vi "DN4_BufferedAO_SetData.vi"(7 "data in(DDT)":dynamicdata(waveform), 8 "error in (no error)":errorcluster, 9 "count":i32, 11 "Task ID":u32) -> (0 "error out":errorcluster, 2 "remaining count":i32, 3 "Task ID":u32)   [LabVIEW 2009]
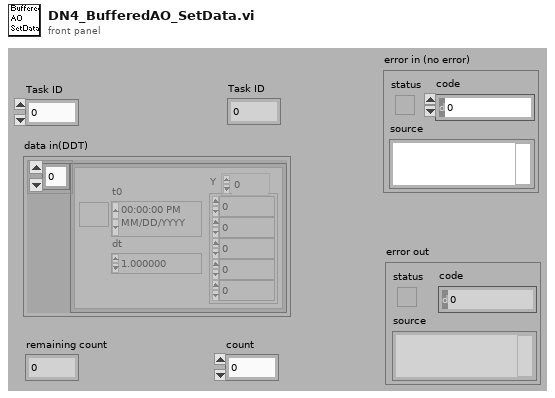
[diagram p1: front panel]
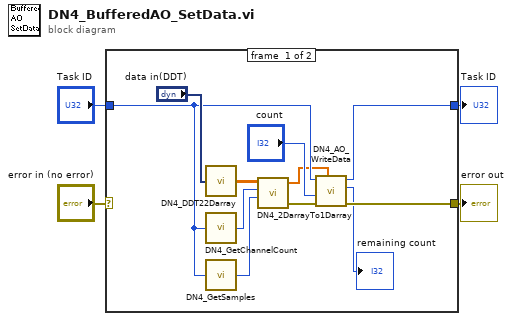
[diagram p0: block diagram]
diagram:
  n1 = case shown="No Error" "error in (no error)" {
    selector: "error in (no error)" -> [_ w17]
    tunnel: [w10 w16] -> w3
    tunnel: [w9 w17] -> w2
    tunnel: "Task ID" -> [w8 w16]
    frame #0 {
      n2 = call <userlib>:"DN4_DDT22Darray.vi"("data"="data in(DDT)") -> ("Array"=w14:dbl[][])
      n3 = call <userlib>:"DN4_GetChannelCount.vi"("Task ID"=w8) -> ("return type"=w13:i32)
      n4 = call <userlib>:"DN4_GetSamples.vi"("Task ID"=w8) -> ("samples"=w12:i32)
      n5 = call <userlib>:"DN4_2DarrayTo1Darray.vi"("samples"=w12, "channel count"=w13, "2Darray"=w14) -> ("error out"=w11:errorcluster, "1Darray"=w6:dbl[])  [unwired: 1 in, 1 out]
      n6 = call <userlib>:"DN4_AO_WriteData.vi"("data"=w6, "error IO"=w11, "count"="count", "Task ID"=w8) -> ("error out"=w9:errorcluster, "remaining count"=→"remaining count":i32, "Task ID"=w10:u32)  [unwired: 1 in, 4 out]
    }
    frame #1 {
    }
  }
  "Task ID" <- w3
  "error out" <- w2
